vi "Deembedding RFSG.vi"(8 "error in":errorcluster, 11 "RFSG Settings":T1={"RFSG Name"="5842_0", "RFSG Port"="", "Attenuation"={"Mode"=enum."Constant Attenuation", "Contant Attenuation"={"RFSG External Attenuation (dB)"=2.0}, "s2p File"={"RFSG S-parameters Orientation"=24000, "RFSG Attenuation s2p Path Name"="", "RFSG s2p File Path"=path ""}}} {"Attenuation"."s2p File"."RFSG S-parameters Orientation" items=["Port1 Towards DUT"=24000, "Port2 Towards DUT"=24001]; "Attenuation"."Contant Attenuation"."RFSG External Attenuation (dB)" format="%.2f"}) -> (0 "error out":errorcluster, 3 "IVI Refnum out":refnum<k15>)   [LabVIEW 2023]
uses:
  RFsg Config.ctl
  <instrlib>/niRFSG/niRFSG.llb/niRFSG Create De-embedding S-parameter Table (S2P file).vi
  <instrlib>/niRFSG/niRFSG.llb/niRFSG Configure De-embedding Table Interpolation (Linear).vi
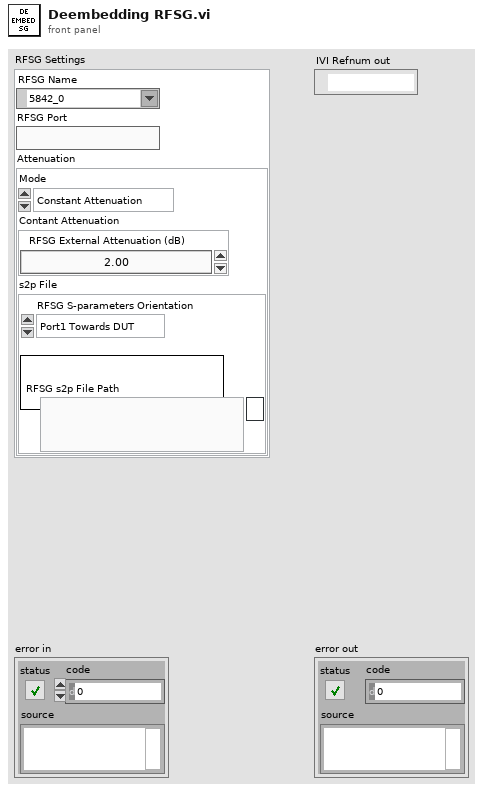
[diagram p1: front panel]
types:
  T1 = typedef "RFsg Config.ctl" = cluster{"RFSG Name":refnum<k15>, "RFSG Port":string, "Attenuation":cluster{"Mode":enum32{"<None>", "Constant Attenuation", "s2p File"}, "Contant Attenuation":cluster{"RFSG External Attenuation (dB)":dbl}, "s2p File":cluster{"RFSG S-parameters Orientation":i32, "RFSG Attenuation s2p Path Name":string, "RFSG s2p File Path":path}}}
  T2 = enum32{"<None>", "Constant Attenuation", "s2p File"}
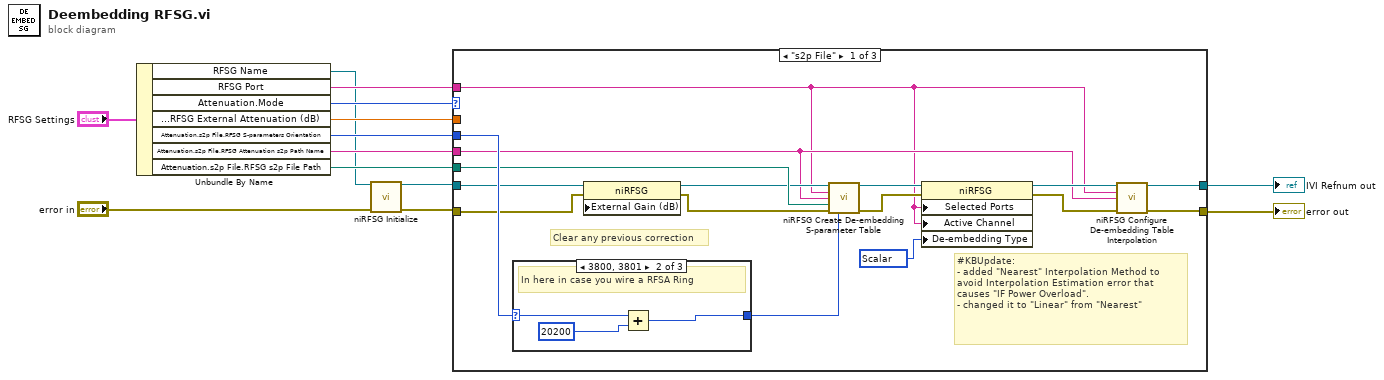
[diagram p0: block diagram]
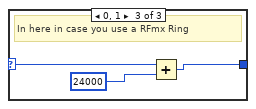
[diagram p3: hidden frame]
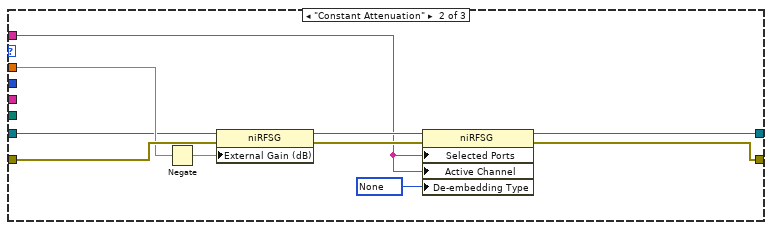
[diagram p4: hidden frame]
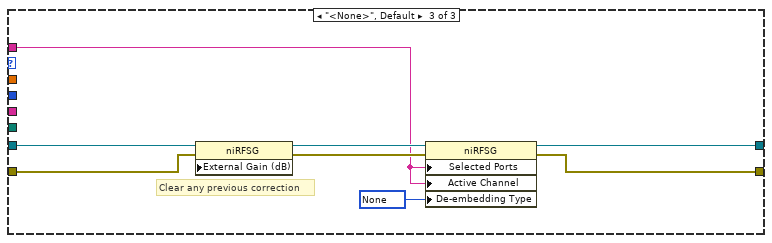
[diagram p5: hidden frame]
diagram:
  n1 = Unbundle By Name("RFSG Settings") -> ("RFSG Name"=w6:refnum<k15>, "RFSG Port"=w12:string, "Attenuation.Mode"=w7:T2, "Attenuation.Contant Attenuation.RFSG External Attenuation (dB)"=w11:dbl, "Attenuation.s2p File.RFSG S-parameters Orientation"=w9:i32, "Attenuation.s2p File.RFSG Attenuation s2p Path Name"=w8:string, "Attenuation.s2p File.RFSG s2p File Path"=w10:path)
  n2 = call <instrlib>:"niRFSG Initialize.vi"("resource name"=w6, "error in"="error in") -> ("instrument handle"=w5:refnum<k15>, "error out"=w3:errorcluster)  [unwired: 12 in]
  n3 = case shown="\"s2p File\"" w7 {
    tunnel: w3 -> [w21 w46 w50]
    tunnel: [w17 w38 w54] -> w2
    tunnel: [w16 w37 w53] -> w1
    tunnel: w9 -> [w26 _ _]
    tunnel: w12 -> [w14 w39 w47]
    tunnel: w11 -> [_ w44 _]
    tunnel: w5 -> [w22 w43 w52]
    tunnel: w10 -> [w25 _ _]
    tunnel: w8 -> [w15 _ _]
    frame "s2p File" {
      w29 = 25001 items=["None"=25000, "Scalar"=25001, "Vector"=25002] ("De-embedding:Type")
      # "#KBUpdate:\n- added \"Nearest\" Interpolation Method to avoid Interpolation Estimation error that causes \"IF Power Overload\".\n- changed it to \"Linear\" from \"Nearest\""
      # "Clear any previous correction"
      n4 = case shown="3800, 3801" w26 {
        selector: w26 -> [w30 w33 w36]
        tunnel: [w30 w31 w35] -> w20
        frame 24000, 24001, Default {
          # "Expected value from API (used a ring)"
        }
        frame 3800, 3801 {
          # "In here in case you wire a RFSA Ring"
          n5 = Add(x=w33, y=20200) -> (x+y=w31:i32)
        }
        frame 0, 1 {
          # "In here in case you use a RFmx Ring"
          n6 = Add(x=w36, y=24000) -> (x+y=w35:i32)
        }
      }
      n7 = property class="niRFSG" props=["External Gain (dB)"](reference=w22, error in=w21) -> (reference out=w24:refnum<k15>, error out=w23:errorcluster)  [unwired: 1 in]
      n8 = call-poly <instrlib>:"niRFSG Create De-embedding S-parameter Table.vi"("instrument handle"=w24, "port"=w14, "table name"=w15, "S2P file path"=w25, "error in"=w23, "S-parameters orientation"=w20) -> ("instrument handle out"=w28:refnum<k15>, "error out"=w27:errorcluster)  [unwired: 8 in]
      n9 = property class="niRFSG"(reference=w28, error in=w27, "Selected Ports"=w14, "Active Channel"=w14, "De-embedding Type"=w29) -> (reference out=w19:refnum<k15>, error out=w18:errorcluster)
      n10 = call-poly <instrlib>:"niRFSG Configure De-embedding Table Interpolation.vi"("instrument handle"=w19, "port"=w14, "table name"=w15, "error in"=w18) -> ("instrument handle out"=w17:refnum<k15>, "error out"=w16:errorcluster)  [unwired: 10 in]
    }
    frame "Constant Attenuation" {
      w42 = 25000 items=["None"=25000, "Scalar"=25001, "Vector"=25002] ("De-embedding:Type")
      n11 = Negate(x=w44) -> (-x=w45:dbl)
      n12 = property class="niRFSG"(reference=w43, error in=w46, "External Gain (dB)"=w45) -> (reference out=w41:refnum<k15>, error out=w40:errorcluster)
      n13 = property class="niRFSG"(reference=w41, error in=w40, "Selected Ports"=w39, "Active Channel"=w39, "De-embedding Type"=w42) -> (reference out=w38:refnum<k15>, error out=w37:errorcluster)
    }
    frame "<None>", Default {
      w48 = 25000 items=["None"=25000, "Scalar"=25001, "Vector"=25002] ("De-embedding:Type")
      # "Clear any previous correction"
      n14 = property class="niRFSG" props=["External Gain (dB)"](reference=w52, error in=w50) -> (reference out=w51:refnum<k15>, error out=w49:errorcluster)  [unwired: 1 in]
      n15 = property class="niRFSG"(reference=w51, error in=w49, "Selected Ports"=w47, "Active Channel"=w47, "De-embedding Type"=w48) -> (reference out=w54:refnum<k15>, error out=w53:errorcluster)
    }
  }
  "error out" <- w1
  "IVI Refnum out" <- w2
